vi "Register Item.vi"(7 "Owner":refnum<class "UniqueName.lvclass">, 8 "error in (no error)":errorcluster, 10 "New Object Name":string, 11 "Registry in":refnum<data-value>) -> (0 "error out":errorcluster, 2 "New Node":refnum<class "UniqueName.lvclass">, 3 "Registry":refnum<data-value>)   [LabVIEW 2014, in "UniqueName.lvlib" / "NameRegistry.lvclass"]
uses:
  NameRegistry.lvclass
  UniqueNameClass/UniqueName.lvclass
  UniqueNameClass/UniqueName.lvclass/UniqueName.ctl
  NameRegistry.lvclass/NameRegistry.ctl
  UniquenessCriteria/UniquenessCriteria.lvclass/UniquenessCriteria.ctl
  UniqueNameClass/Key.ctl
  UniqueNameClass/Write UUID.vi
  RandomStringGenerator/Generate Random String.vi
  Delimiter/DelimiterToStringRepresentation.vi
  <vilib>/Utility/error.llb/Trim Whitespace.vi
  UniquenessCriteria/UniquenessCriteria.lvclass
  NameIncrementAlgorithm/StringIncrement.lvclass
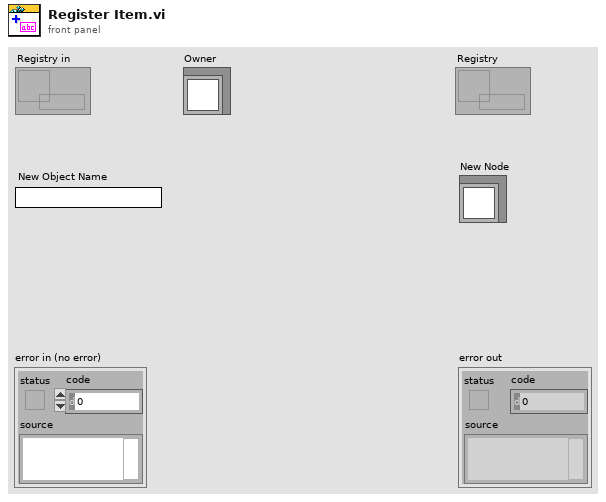
[diagram p1: front panel]
types:
  T1 = typedef "UniqueName.lvlib/UniqueName.lvclass/Key.ctl" = enum16{"Fully Qualified Name", "Unique Name", "Given Name", "Parent Fully Qualified Name"}
  T2 = typedef "UniquenessCriteria.lvclass/Criteria.ctl" = enum16{"Globally-Unique Fully Qualified Name", "Globally-Unique Name"}
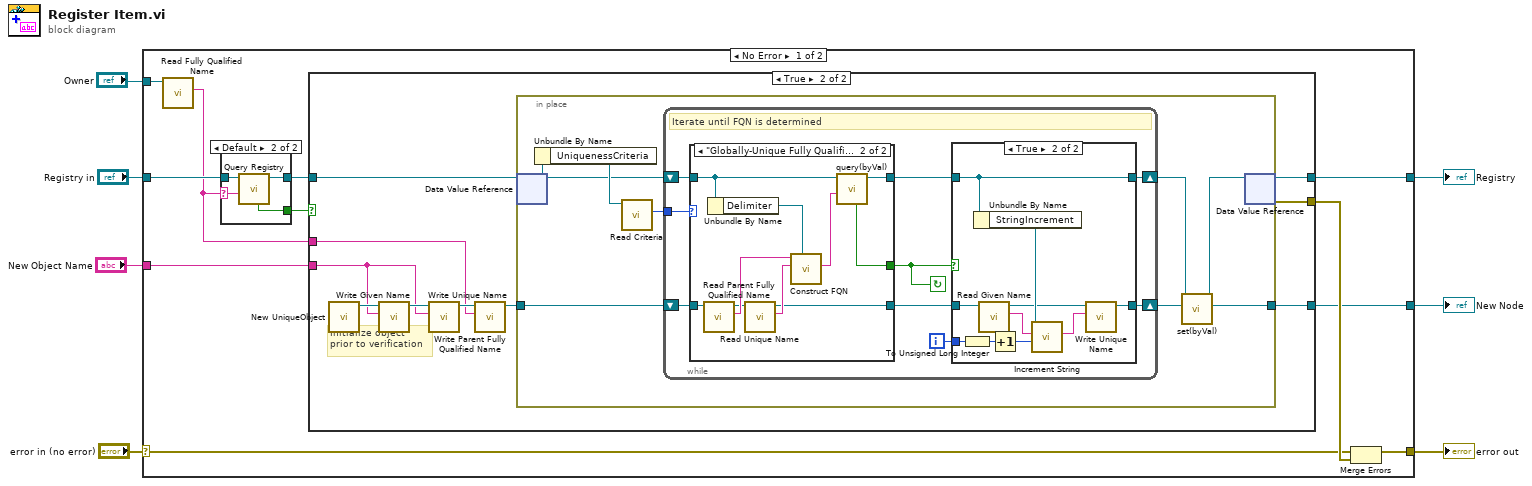
[diagram p0: block diagram]
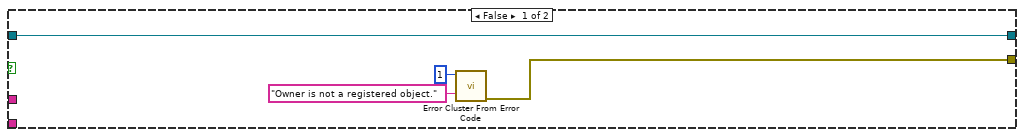
[diagram p2: hidden frame]
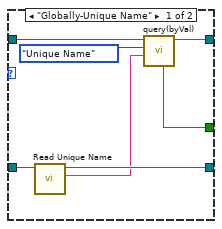
[diagram p4: hidden frame]
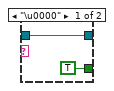
[diagram p5: hidden frame]
diagram:
  n1 = case shown="No Error" "error in (no error)" {
    selector: "error in (no error)" -> [w16 w85]
    tunnel: "Registry in" -> [w14 w86]
    tunnel: [w18 w86] -> w6
    tunnel: [w15 w85] -> w4
    tunnel: "Owner" -> [w9 _]
    tunnel: "New Object Name" -> [w11 _]
    tunnel: [w10 _] -> w2
    frame No Error {
      n2 = call "Read Fully Qualified Name.vi"("UniqueName in"=w9) -> ("Fully Qualified Name"=w8:string)  [unwired: 9 in, 1 out]
      n3 = case shown="Default" w8 {
        selector: w8 -> [_ w82]
        tunnel: w14 -> [w80 w84]
        tunnel: [w80 w83] -> w13
        tunnel: [TRUE ("found?") w81] -> w12
        frame "\u0000" {
        }
        frame Default {
          n4 = call "Query Registry.vi"("Search string"=w82, "Registry in"=w84) -> ("Registry"=w83:refnum<data-value>, "found?"=w81:bool)  [unwired: 5 in, 3 out]
        }
      }
      n5 = case shown="True" w12 {
        tunnel: [w22 w32] -> w18
        tunnel: [w20 w31] -> w17
        tunnel: w13 -> [w22 w25]
        tunnel: w11 -> [_ w27]
        tunnel: w8 -> [_ w26]
        tunnel: [_ w23] -> w10
        frame False {
          n6 = call <vilib>:"Error Cluster From Error Code.vi"("error message (\"\")"="Owner is not a registered object." ("error message (\"\")"), "error code (0)"=1) -> ("error out"=w20:errorcluster)  [unwired: 7 in]
        }
        frame True {
          # "Initialize object\nprior to verification"
          n7 = call "New UniqueObject.vi"() -> ("UniqueName out"=w30:refnum<class "UniqueName.lvclass">)  [unwired: 11 in]
          n8 = call "Write Given Name.vi"("Given Name"=w27, "UniqueName in"=w30) -> ("UniqueName out"=w28:refnum<class "UniqueName.lvclass">)  [unwired: 9 in]
          n9 = call "Write Unique Name.vi"("Unique Name"=w27, "UniqueName in"=w28) -> ("UniqueName out"=w29:refnum<class "UniqueName.lvclass">)  [unwired: 9 in]
          n10 = call "Write Parent Fully Qualified Name.vi"("Parent Fully Qualified Name"=w26, "UniqueName in"=w29) -> ("UniqueName out"=w24:refnum<class "UniqueName.lvclass">)  [unwired: 9 in]
          n11 = in-place {
            in-place-border: w24 -> [w38]
            in-place-border: [w35] -> w23
            n12 = in-place-dvr #1(w25) -> (w37:refnum<class "NameRegistry.lvclass">)  [unwired: 1 out]
            n13 = Unbundle By Name(w37) -> ("UniquenessCriteria"=w40:refnum<class "UniquenessCriteria.lvclass">)
            n14 = call "Read Criteria.vi"("UniquenessCriteria in"=w40) -> ("Criteria"=w39:T2)  [unwired: 9 in, 1 out]
            n15 = while {
              tunnel: w39 -> [w49]
              shift-right: [w47] -> w36
              shift-left: w38 -> [w46]
              shift-right: [w41] -> w34
              shift-left: w37 -> [w43]
              i -> [w44]
              stop <- w45 continue-if-true
              # "Iterate until FQN is determined"
              n16 = case shown="\"Globally-Unique Fully Qualified Name\"" w49 {
                tunnel: [w65 w72] -> w45
                tunnel: w46 -> [w68 w76]
                tunnel: [w67 w74] -> w48
                tunnel: w43 -> [w66 w70]
                tunnel: [w62 w71] -> w42
                frame "Globally-Unique Name" {
                  n17 = call "Read Unique Name.vi"("UniqueName in"=w68) -> ("Unique Name"=w63:string, "UniqueName out"=w67:refnum<class "UniqueName.lvclass">)  [unwired: 9 in]
                  n18 = call "query(byVal).vi"("Search string"=w63, "Search Key (FQN)"=Key."Unique Name" ("Key (FQN)"), "Instance"=w66) -> ("Instance"=w62:refnum<class "NameRegistry.lvclass">, "found?"=w65:bool)  [unwired: 5 in, 2 out]
                }
                frame "Globally-Unique Fully Qualified Name" {
                  n19 = call "Read Parent Fully Qualified Name.vi"("UniqueName in"=w76) -> ("Parent Fully Qualified Name"=w78:string, "UniqueName out"=w75:refnum<class "UniqueName.lvclass">)  [unwired: 9 in]
                  n20 = Unbundle By Name(w70) -> ("Delimiter"=w69:refnum<class "Delimiter.lvclass">)
                  n21 = call "Read Unique Name.vi"("UniqueName in"=w75) -> ("Unique Name"=w77:string, "UniqueName out"=w74:refnum<class "UniqueName.lvclass">)  [unwired: 9 in]
                  n22 = call "Construct FQN.vi"("Delimiter"=w69, "Name"=w77, "Parent FQN"=w78) -> ("FQN"=w73:string)  [unwired: 8 in]
                  n23 = call "query(byVal).vi"("Search string"=w73, "Instance"=w70) -> ("Instance"=w71:refnum<class "NameRegistry.lvclass">, "found?"=w72:bool)  [unwired: 6 in, 2 out]
                }
              }
              n24 = case shown="True" w45 {
                tunnel: w48 -> [w51 w56]
                tunnel: [w51 w61] -> w47
                tunnel: w44 -> [_ w59]
                tunnel: w42 -> [w50 w58]
                tunnel: [w50 w58] -> w41
                frame False {
                  # "Name already unique"
                }
                frame True {
                  n25 = To Unsigned Long Integer(number=w59) -> (unsigned 32bit integer=w53:u32)
                  n26 = Unbundle By Name(w58) -> ("StringIncrement"=w57:refnum<class "StringIncrement.lvclass">)
                  n27 = call "Read Given Name.vi"("UniqueName in"=w56) -> ("Given Name"=w55:string, "UniqueName out"=w54:refnum<class "UniqueName.lvclass">)  [unwired: 9 in]
                  n28 = Increment(x=w53) -> (x+1=w52:u32)
                  n29 = call "Increment String.vi"("Numeric"=w52, "Input String"=w55, "StringIncrement"=w57) -> ("Incremented String"=w60:string)  [unwired: 8 in]
                  n30 = call "Write Unique Name.vi"("Unique Name"=w60, "UniqueName in"=w54) -> ("UniqueName out"=w61:refnum<class "UniqueName.lvclass">)  [unwired: 9 in]
                }
              }
            }
            n31 = call "set(byVal).vi"("UniqueName in"=w36, "NameRegistry in"=w34) -> ("UniqueName out"=w35:refnum<class "UniqueName.lvclass">, "NameRegistry out"=w33:refnum<class "NameRegistry.lvclass">)  [unwired: 7 in, 1 out]
            n32 = in-place-dvr #1(w33) -> (w32:refnum<data-value>, w31:errorcluster)
          }
        }
      }
      n33 = Merge Errors(w16, w17) -> (w15:errorcluster)
    }
    frame Error {
    }
  }
  "error out" <- w4
  "Registry" <- w6
  "New Node" <- w2
